vi "CaLabPut_Main_Initialized.vi"(0 "CA Lab data":T2, 1 "Data Type":i32, 5 "Values [String]":string[][](array[string]), 7 "Values[Double]":dbl[][](array[numeric]), 9 "Values [I64]":i64[][](array[numeric]), 11 "Error in (no error)":errorcluster) -> (4 "PV Names (dup)":string[](array[string]), 6 "Status":bool, 10 "PV Errors":errorcluster[](array[cluster]), 15 "Error out":errorcluster)   [LabVIEW 2018]
uses:
  <userlib>/caLab/PV Info.ctl
  <userlib>/caLab/lib/caLab.dll
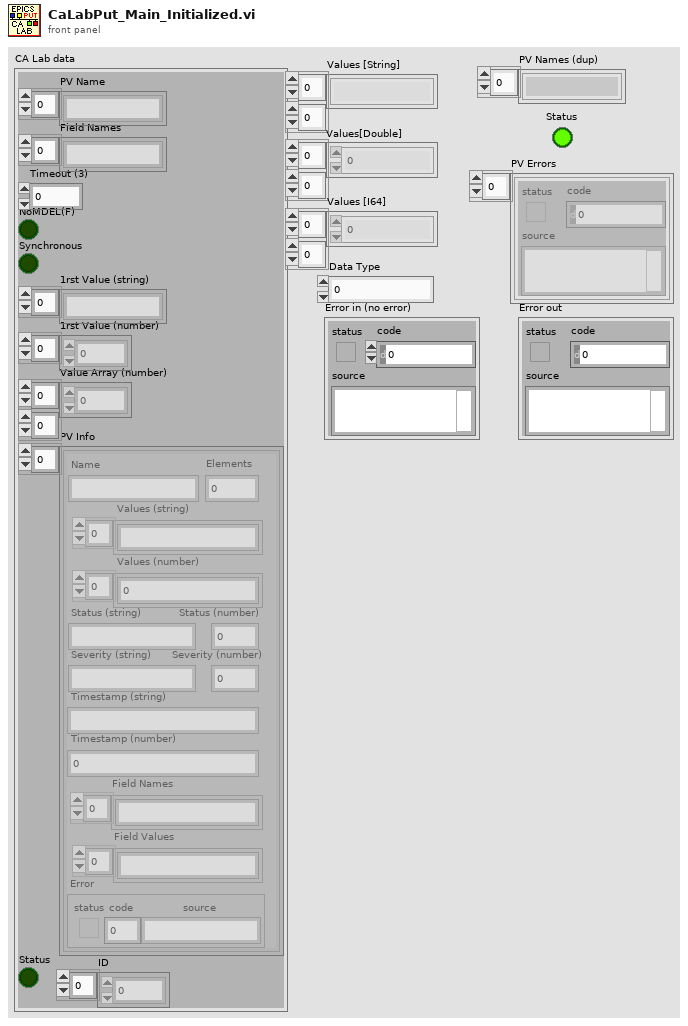
[diagram p1: front panel]
types:
  T1 = typedef "PV Info.ctl" = cluster{"Name":string, "Elements":i32, "Values (string)":string[], "Values (number)":dbl[], "Status (string)":string, "Status (number)":i16, "Severity (string)":string, "Severity (number)":i16, "Timestamp (string)":string, "Timestamp (number)":i32, "Field Names":string[], "Field Values":string[], "Error":errorcluster}
  T2 = cluster{"PV Name":string[], "Field Names":string[], "Timeout (3)":dbl, "NoMDEL(F)":bool, "Synchronous":bool, "1rst Value (string)":string[], "1rst Value (number)":dbl[], "Value Array (number)":dbl[][], "PV Info":T1[], "Status":bool, "ID":u64[]}
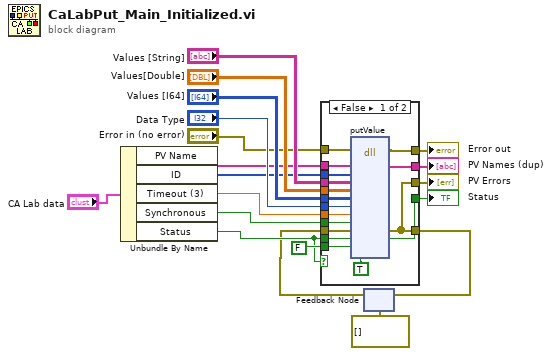
[diagram p0: block diagram]
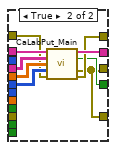
[diagram p2: hidden frame]
diagram:
  n1 = Unbundle By Name("CA Lab data") -> ("PV Name"=w13:string[], "ID"=w12:u64[], "Timeout (3)"=w11:dbl, "Synchronous"=w10:bool, "Status"=w4:bool)
  n2 = feedback #1(errorcluster[] []) -> (w2:errorcluster[])
  n3 = case shown="False" w4 {
    tunnel: "Values [String]" -> [w36 w44]
    tunnel: "Values[Double]" -> [w35 w43]
    tunnel: "Values [I64]" -> [w34 w42]
    tunnel: "Data Type" -> [w33 _]
    tunnel: w2 -> [w32 _]
    tunnel: FALSE ("FirstCall") -> [w31 _]
    tunnel: w13 -> [w30 w45]
    tunnel: w12 -> [w29 _]
    tunnel: w11 -> [w28 _]
    tunnel: w10 -> [w27 _]
    tunnel: w4 -> [w26 _]
    tunnel: [w25 w39] -> w9
    tunnel: [w24 w40] -> w8
    tunnel: [w20 w37] -> w7
    tunnel: [w23 w38] -> w6
    tunnel: "Error in (no error)" -> [w21 w41]
    tunnel: [w20 w37] -> w3
    frame False {
      n4 = dll-call lib="D:/Program Files (x86)/National Instruments/LabVIEW 2018/user.lib/caLab/lib/calab.dll" fn="putValue" label="caLabPut"(error in=w21, "PVNameArray"=w30, "IndexArray"=w29, "ValueArrayString"=w36, "ValueArrayDoubleFloat"=w35, "ValueArrayI64"=w34, "DataType"=w33, "Timeout"=w28, "Synchronous"=w27, "ErrorArray"=w32, "Status"=w26, "FirstCall"=w31, "IsInitialized"=TRUE ("FirstCall")) -> (error out=w25:errorcluster, "PVNameArray"=w24:string[], "ErrorArray"=w20:errorcluster[], "Status"=w23:bool)  [unwired: 9 in, 4 out]
    }
    frame True {
      n5 = call <userlib>:"CaLabPut_Main.vi"("PV Names"=w45, "Values [String]"=w44, "Values [DBL]"=w43, "Values [I64]"=w42, "Error in (no error)"=w41) -> ("PV Names (dup)"=w40:string[], "Status"=w38:bool, "PV Errors"=w37:errorcluster[], "Error out"=w39:errorcluster)  [unwired: 7 in]
    }
  }
  "PV Errors" <- w7
  "Status" <- w6
  "Error out" <- w9
  "PV Names (dup)" <- w8
  n6 = feedback-in #1(w3) -> ()
